vi "Retrieve SubComponent Parameter.vi"(5 "Component ID":u8, 7 "FPGA Interface":refnum<class "FPGA Interface.lvclass">, 8 "error in (no error)":errorcluster, 10 "Parameter":string, 11 "1553 SubComponent in":refnum<class "1553 SubComponent.lvclass">) -> (0 "error out":errorcluster, 3 "1553 SubComponent out":refnum<class "1553 SubComponent.lvclass">)   [LabVIEW 2020, in "BCI-1553 API.lvlib" / "1553 SubComponent.lvclass"]
doc: "Retrieves a specific parameter from the 1553 Session component. A read must be called after this to retrieve the specific parameter values."
uses:
  1553 SubComponent.lvclass
  Dependencies/FPGA Interface/FPGA Interface.lvclass
  Frames & Messages/TypeDefs/Parameter Table Data.ctl
  Frames & Messages/TypeDefs/Scaling Information.ctl
  1553 SubComponent.lvclass/1553 SubComponent.ctl
  Dependencies/Registry/Registry.lvclass/Registry.ctl
  BCI-1553 API.lvlib
  Dependencies/Registry/Registry.lvclass
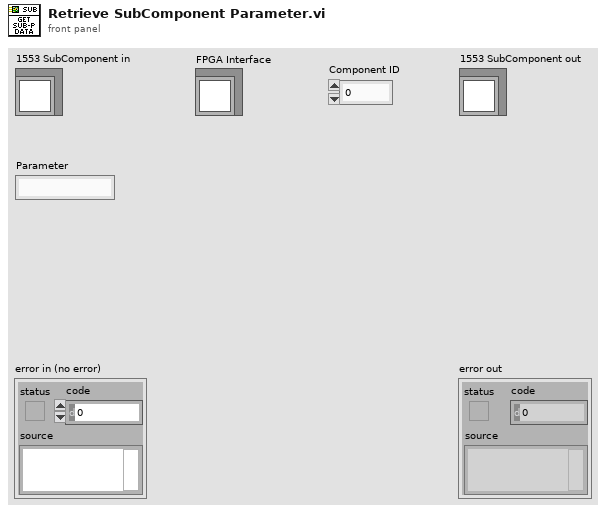
[diagram p1: front panel]
types:
  T1 = typedef "BCI-1553 API.lvlib/Parameter Table Data.ctl" = cluster{"Parameter Name":string, "Base Word":u16, "Address":u16, "Value":u64, "Mask":u16[], "Scaling Info":T2}
  T2 = typedef "BCI-1553 API.lvlib/Scaling Information.ctl" = cluster{"Bit Offset":i32, "Bit Count":i32, "LSB Resolution":dbl, "2's Complement":bool, "Big Endian":bool, "Sign Bit":bool}
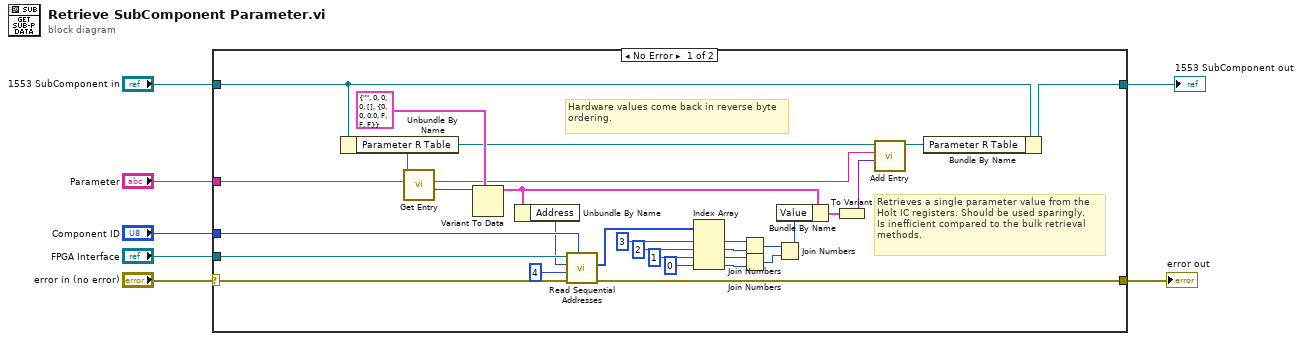
[diagram p0: block diagram]
diagram:
  n1 = case shown="No Error" "error in (no error)" {
    selector: "error in (no error)" -> [w35 w38]
    tunnel: [w32 w38] -> w2
    tunnel: [w30 w37] -> w1
    tunnel: "1553 SubComponent in" -> [w31 w37]
    tunnel: "FPGA Interface" -> [w34 _]
    tunnel: "Component ID" -> [w33 _]
    tunnel: "Parameter" -> [w22 _]
    frame No Error {
      # "Hardware values come back in reverse byte ordering."
      # "Retrieves a single parameter value from the\nHolt IC registers. Should be used sparingly.\nIs inefficient compared to the bulk retrieval\nmethods."
      n2 = Unbundle By Name(w31) -> ("Parameter R Table"=w24:refnum<class "Registry.lvclass">)
      n3 = call "Get Entry.vi"("Key"=w22, "Registry in"=w24) -> ("Value"=w23:variant, "Key Out"=w20:string)  [unwired: 6 in, 2 out]
      n4 = Variant To Data(type=T1 {"Parameter Name"="", "Base Word"=0, "Address"=0, "Value"=0, "Mask"=[], "Scaling Info"={"Bit Offset"=0, "Bit Count"=0, "LSB Resolution"=0.0, "2's Complement"=FALSE, "Big Endian"=FALSE, "Sign Bit"=FALSE}} ("Parameter Table Data"), Variant=w23) -> (data=w27:T1)  [unwired: 1 in, 1 out]
      n5 = Unbundle By Name(w27) -> ("Address"=w29:u16)
      n6 = call-dynamic "Read Sequential Addresses.vi"("Target IC (1-8)"=w33, "error in (no error)"=w35, "Addresses to Read"=u16 4, "Starting Address"=w29, "FPGA Interface in"=w34) -> ("error out"=w32:errorcluster, "Data"=w13:u16[])  [unwired: 5 in]
      n7 = Index Array(array=w13, index #1=3 ("index"), index #2=2 ("index"), index #3=1 ("index"), index #4=0 ("index")) -> (element #1=w16:u16, element #2=w17:u16, element #3=w15:u16, element #4=w14:u16)
      n8 = Join Numbers(hi=w16, lo=w17) -> ((hi.lo)=w18:u32)
      n9 = Join Numbers(hi=w15, lo=w14) -> ((hi.lo)=w19:u32)
      n10 = Join Numbers(hi=w18, lo=w19) -> ((hi.lo)=w12:u64)
      n11 = Bundle By Name(cluster=w27, "Value"=w12) -> (w26:T1)
      n12 = To Variant(anything=w26) -> (Variant=w21:variant)
      n13 = call "Add Entry.vi"("Value"=w21, "Key"=w20, "Registry in"=w24) -> ("Registry out"=w25:refnum<class "Registry.lvclass">)  [unwired: 6 in, 2 out]
      n14 = Bundle By Name(cluster=w31, "Parameter R Table"=w25) -> (w30:refnum<class "1553 SubComponent.lvclass">)
    }
    frame Error {
    }
  }
  "error out" <- w2
  "1553 SubComponent out" <- w1
